vi "Insert Front Panel.vi"(8 "error in (no error)":errorcluster, 9 "Insertion Request Time":timestamp, 10 "Protected Subpanel":T1, 11 "String Type View in":refnum<class "Float Type View.lvclass">) -> (0 "error out":errorcluster, 3 "String Type View out":refnum<class "Float Type View.lvclass">)   [LabVIEW 2017, in "Float Type View.lvclass"]
doc: "<License>\nCopyright © 2017 Composed Systems, LLC | All rights reserved\nwww.composed.io\n\nAuthor: Ethan Stern <ethan.stern@composed.io>\n\nThis software is provided \"AS IS\" WITHOUT WARRANTIES, either express or implied, AND IS FOR EDUCATIONAL PURPOSES ONLY.\n</License>"
uses:
  Float Type View.lvclass
  IAttribute Data Type View/IAttribute Data Type View.lvclass
  <vilib>/gpm_packages/@cs/mva-viewable/Source/IViewable/ProtectedSubpanel/Protected Subpanel Reference.ctl
  <vilib>/gpm_packages/@cs/mva-viewable/Source/IViewable/ProtectedSubpanel/ProtectedSubpanel.lvclass
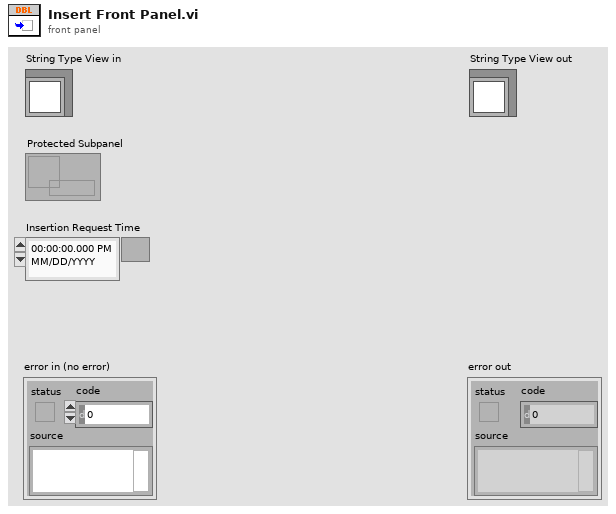
[diagram p1: front panel]
types:
  T1 = typedef "IViewable.lvlib/ProtectedSubpanel.lvclass/Protected Subpanel Reference.ctl" = refnum<data-value>
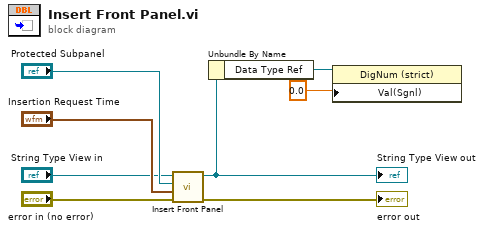
[diagram p0: block diagram]
diagram:
  n1 = call-parent "Insert Front Panel.vi"("error in (no error)"="error in (no error)", "Insertion Request Time"="Insertion Request Time", "Protected Subpanel"="Protected Subpanel", "IViewable in"="String Type View in") -> ("error out"=→"error out":errorcluster, "IViewable out"=w3:refnum<class "Float Type View.lvclass">)  [unwired: 6 in]
  "String Type View out" <- w3
  n2 = Unbundle By Name(w3) -> ("Data Type Ref"=w2:refnum<vi>)
  n3 = property class="DigNum (strict)"(reference=w2, "Val(Sgnl)"=0.0) -> ()  [unwired: 1 in, 2 out]
